vi "Get Module Info (Scan Mode).vi"(8 "error in":errorcluster, 11 "Session in":refnum<k21>="localhost") -> (0 "error out":errorcluster, 2 "Module Information":T1[](array[typedef]) {"Module Code" format="%.0x"}, 3 "Session out":refnum<k21>="localhost")   [LabVIEW 2015]
uses:
  <resource>/objmgr/ni.var.rc
  <vilib>/regexp/Match Regular Expression.xnode
  Controls/ModuleInformation.ctl
  <resource>/objmgr/nisysapi.rc
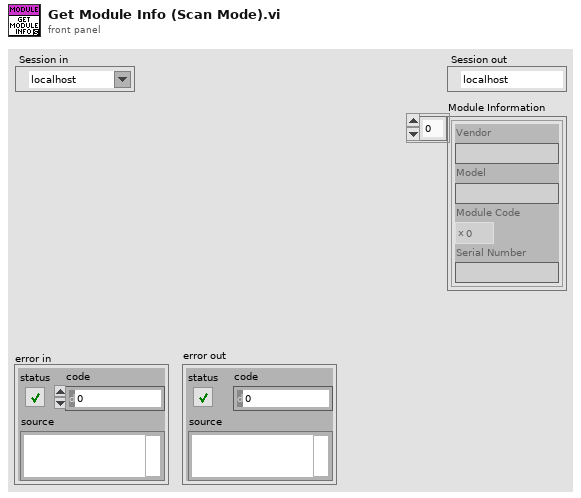
[diagram p1: front panel]
types:
  T1 = typedef "RT Management.lvlib/Module Detection.lvclass/ModuleInformation.ctl" = cluster{"Vendor":string, "Model":string, "Module Code":u32, "Serial Number":string}
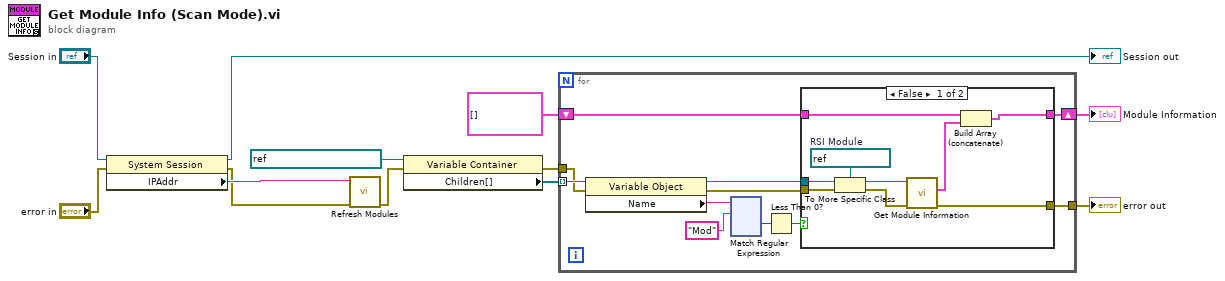
[diagram p0: block diagram]
diagram:
  n1 = property class="System Session"(reference="Session in", error in="error in") -> (reference out=→"Session out":refnum<k21>, error out=w2:errorcluster, "IPAddr"=w4:string)
  n2 = call <vilib>:"Refresh Modules.vi"("error in (no error)"=w2, "target address (localhost)"=w4) -> ("error out"=w9:errorcluster)  [unwired: 9 in]
  n3 = property class="Variable Container"(reference=refnum<k21> "ni.var.io://localhost" ("container refnum in"), error in=w9) -> (error out=w11:errorcluster, "Children[]"=w10:refnum<k21>[])  [unwired: 1 out]
  n4 = for {
    tunnel: w10 -> [w16] mode=indexing
    tunnel: w11 -> [w14]
    tunnel: [w20] -> w7
    shift-right: [w19] -> w8
    shift-left: T1[] [] -> [w18]
    n5 = property class="Variable Object"(reference=w16, error in=w14) -> (reference out=w15:refnum<k21>, error out=w13:errorcluster, "Name"=w21:string)
    n6 = xnode "Match Regular Expression"("input string"=w21, "regular expression"="Mod") -> ("offset past match"=w23:i32)  [unwired: 4 in, 4 out]
    n7 = Less Than 0?(x=w23) -> (x < 0?=w17:bool)
    n8 = case shown="False" w17 {
      tunnel: w13 -> [w31 w33]
      tunnel: w15 -> [w30 _]
      tunnel: [w24 w33] -> w20
      tunnel: [w29 w34] -> w19
      tunnel: w18 -> [w28 w34]
      frame False {
        w32 = refnum<k21> refnum  # RSI Module
        n9 = To More Specific Class(target class=w32, reference=w30, error in=w31) -> (specific class reference=w27:refnum<k21>, error out=w26:errorcluster)
        n10 = call "Get Module Information.vi"("error in"=w26, "Module reference"=w27) -> ("error out"=w24:errorcluster, "Module Information"=w25:T1)  [unwired: 8 in]
        n11 = Build Array (concatenate)(w28, w25) -> (w29:T1[])
      }
      frame True {
        # "The Variable Object is not a module"
      }
    }
  }
  "error out" <- w7
  "Module Information" <- w8
